vi "Write Vehicle Out of Position.vi"(8 "error in (no error)":errorcluster, 10 "Vehicle Out of Position":bool, 11 "Sim Wash Display Console in":refnum<class "Sim Wash Display Console.lvclass">) -> (0 "error out":errorcluster, 3 "Sim Wash Display Console out":refnum<class "Sim Wash Display Console.lvclass">)   [LabVIEW 2019, in "Sim Wash Display Console.lvlib" / "Sim Wash Display Console.lvclass"]
uses:
  Sim Wash Display Console.lvclass
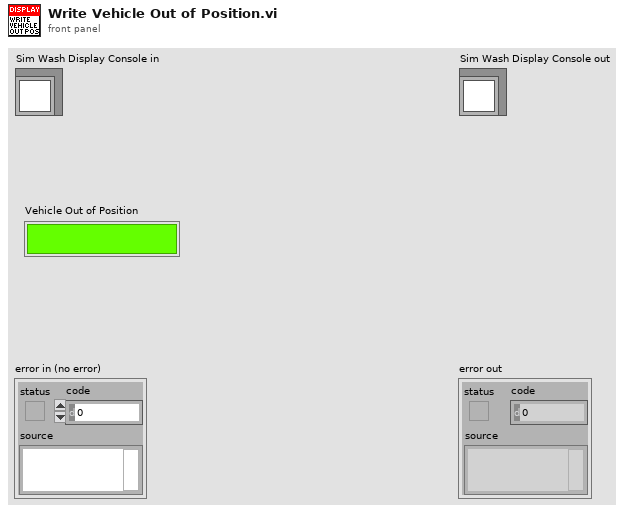
[diagram p1: front panel]
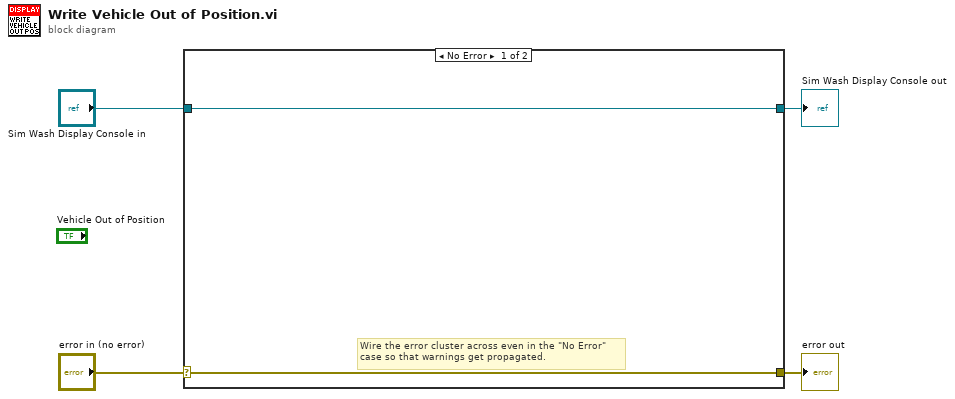
[diagram p0: block diagram]
diagram:
  n1 = case shown="No Error" "error in (no error)" {
    selector: "error in (no error)" -> [w5 w8]
    tunnel: [w5 w8] -> w3
    tunnel: [w6 w7] -> w1
    tunnel: "Sim Wash Display Console in" -> [w6 w7]
    frame No Error {
      # "Wire the error cluster across even in the \"No Error\"\ncase so that warnings get propagated."
    }
    frame Error {
    }
  }
  "error out" <- w3
  "Sim Wash Display Console out" <- w1
